vi "SetDcOffset.vi"(8 "error in (no error)":errorcluster, 9 "FPGA Setting":T1=enum."DC_offs 1", 10 "DC offset":dbl caption="DC offset\nChannel 1", 11 "FpgaRef5782 in":refnum<class "FpgaRef5782.lvclass">) -> (0 "error out":errorcluster, 3 "FpgaRef5782 in":refnum<class "FpgaRef5782.lvclass">)   [LabVIEW 2018, in "FpgaRef5782.lvclass"]
uses:
  FpgaRef5782.lvclass
  FPGA/fpga_settings.ctl
  <vilib>/rvi/FXPMathLib/FxpInterpret/XNode/nifxpmath_Interpret.xnode
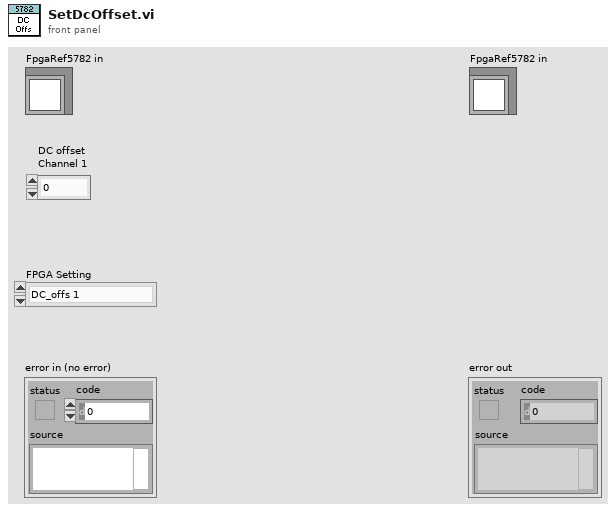
[diagram p1: front panel]
types:
  T1 = typedef "fpga_settings.ctl" = enum16{"Feedback Enable", "New FIR coeffs", "FIR shift", "Enable filter", "Set Downsample", "Downsample", "CIC Gain", "Record length", "Trigger samples", "Quiet time", "a_am", "b_am", "Use fixed delay", "fixed sin_fi", "fixed cos_fi", "Ki*Tau", "Kp", "Kd_Tau", "Fi_start", "Fi_delta", "DC_offs 0", "DC_offs 1", "DC_offs 2", "DC_offs 3", "Ki*Tau am", "Kp am", "Kd_Tau am", "Feedback AM", "Trigger delay", "Feedback delay", "Setpoint enable", "Beam enable", "Samples to acquire", "Cavity Enable", "Cavity C1", "Cavity C2", "Cavity C3", "Cavity C4", "Cavity C5", "Input delay", "Ki*Tau Q", "Kp Q", "Kd_Tau Q", "Adaptive FF enable", "Feedforward a0", "Feedforward b0", "FF src adress", "FF dest adress", "Output scale", "Input scale", "Host scale"}
  T2 = typedef "settingsFPGAref.ctl" = refnum<k20>
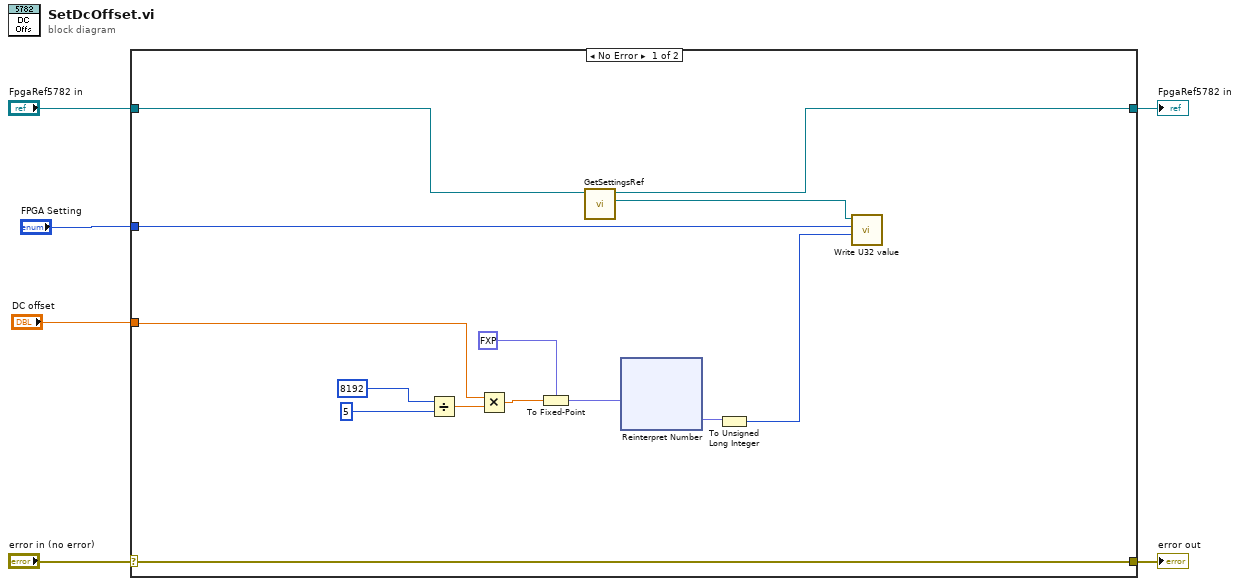
[diagram p0: block diagram]
diagram:
  n1 = case shown="No Error" "error in (no error)" {
    selector: "error in (no error)" -> [w20 w22]
    tunnel: [w20 w22] -> w5
    tunnel: [w18 w21] -> w3
    tunnel: "FpgaRef5782 in" -> [w17 w21]
    tunnel: "DC offset" -> [w8 _]
    tunnel: "FPGA Setting" -> [w16 _]
    frame No Error {
      n2 = Divide(x=8192, y=5) -> (x/y=w14:dbl)
      n3 = Multiply(x=w8, y=w14) -> (x*y=w9:dbl)
      n4 = To Fixed-Point(fixed-point type=fxp<+/-,32,14> 0.0 ("y 2"), number=w9) -> (fixed-point=w11:fxp<+/-,32,14>)
      n5 = call-dynamic "GetSettingsRef.vi"("FpgaRef5782 In"=w17) -> ("Settings FPGA ref"=w19:T2, "FpgaRef5782 Out"=w18:refnum<class "FpgaRef5782.lvclass">)  [unwired: 8 in, 1 out]
      n6 = xnode "Reinterpret Number"("x"=w11) -> ("y"=w10:fxp<+,32,32>)
      n7 = To Unsigned Long Integer(number=w10) -> (unsigned 32bit integer=w7:u32)
      n8 = call "Write U32 value.vi"("value"=w7, "FPGA Setting"=w16, "FPGA ref"=w19) -> ()  [unwired: 7 in, 2 out]
    }
    frame Error {
    }
  }
  "error out" <- w5
  "FpgaRef5782 in" <- w3
